vi "searchDataType.vi"(8 "error in (no error)":errorcluster, 10 "regExpr":string, 11 "LibReader in":refnum<class "LibReader.lvclass">) -> (0 "error out":errorcluster, 2 "pathDataType":path, 3 "LibReader out":refnum<class "LibReader.lvclass">)   [LabVIEW 2018, in "LibReader.lvclass"]
doc: "Search the data type."
uses:
  LibReader.lvclass
  LibReader.lvclass/LibReader.ctl
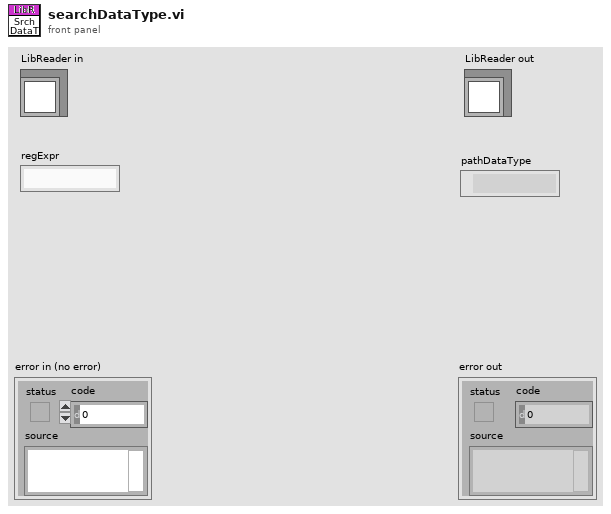
[diagram p1: front panel]
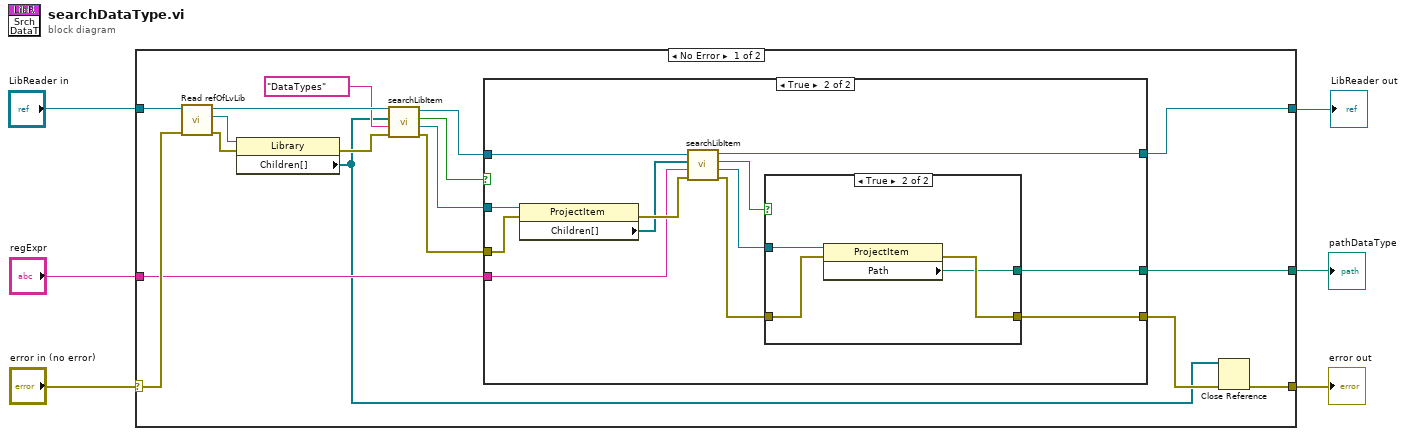
[diagram p0: block diagram]
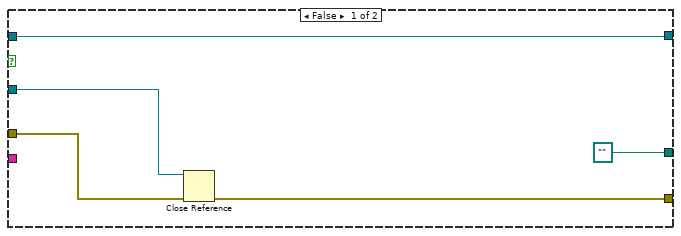
[diagram p2: hidden frame]
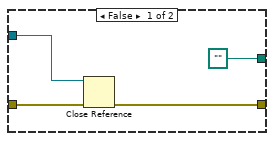
[diagram p3: hidden frame]
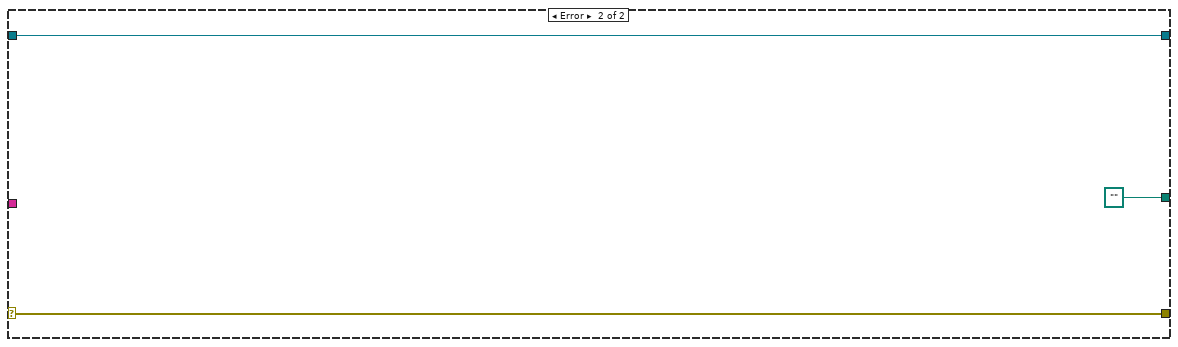
[diagram p4: hidden frame]
diagram:
  n1 = case shown="No Error" "error in (no error)" {
    selector: "error in (no error)" -> [w21 w51]
    tunnel: [w9 w51] -> w5
    tunnel: [w11 w50] -> w2
    tunnel: "LibReader in" -> [w23 w50]
    tunnel: "regExpr" -> [w12 _]
    tunnel: [w10 path "" ("Path")] -> w3
    frame No Error {
      n2 = call "Read refOfLvLib.vi"("error in (no error)"=w21, "LibReader in"=w23) -> ("error out"=w19:errorcluster, "refOfLvLib"=w20:refnum<vi>, "LibReader out"=w22:refnum<class "LibReader.lvclass">)  [unwired: 7 in]
      n3 = property class="Library"(reference=w20, error in=w19) -> (error out=w18:errorcluster, "Children[]"=w7:refnum<vi>[])  [unwired: 1 out]
      n4 = call "searchLibItem.vi"("error in (no error)"=w18, "regExpr"="DataTypes", "Owned Items[]"=w7, "LibReader in"=w22) -> ("error out"=w14:errorcluster, "ProjectItem Refnum"=w15:refnum<vi>, "found"=w16:bool, "LibReader out"=w13:refnum<class "LibReader.lvclass">)  [unwired: 4 in]
      n5 = case shown="True" w16 {
        tunnel: w15 -> [w26 w39]
        tunnel: w14 -> [w25 w38]
        tunnel: w13 -> [w28 w40]
        tunnel: w12 -> [_ w36]
        tunnel: [w28 w35] -> w11
        tunnel: [w24 w29] -> w8
        tunnel: [path "" ("Path") w32] -> w10
        frame False {
          n6 = Close Reference(reference=w26, error in (no error)=w25) -> (error out=w24:errorcluster)
        }
        frame True {
          n7 = property class="ProjectItem"(reference=w39, error in=w38) -> (error out=w37:errorcluster, "Children[]"=w30:refnum<vi>[])  [unwired: 1 out]
          n8 = call "searchLibItem.vi"("error in (no error)"=w37, "regExpr"=w36, "Owned Items[]"=w30, "LibReader in"=w40) -> ("error out"=w33:errorcluster, "ProjectItem Refnum"=w34:refnum<vi>, "found"=w31:bool, "LibReader out"=w35:refnum<class "LibReader.lvclass">)  [unwired: 4 in]
          n9 = case shown="True" w31 {
            tunnel: w34 -> [w43 w48]
            tunnel: w33 -> [w42 w47]
            tunnel: [w41 w46] -> w29
            tunnel: [path "" ("Path") w45] -> w32
            frame False {
              n10 = Close Reference(reference=w43, error in (no error)=w42) -> (error out=w41:errorcluster)
            }
            frame True {
              n11 = property class="ProjectItem"(reference=w48, error in=w47) -> (error out=w46:errorcluster, "Path"=w45:path)  [unwired: 1 out]
            }
          }
        }
      }
      n12 = Close Reference(reference=w7, error in (no error)=w8) -> (error out=w9:errorcluster)
    }
    frame Error {
    }
  }
  "error out" <- w5
  "LibReader out" <- w2
  "pathDataType" <- w3
